vi "2_InsertQueue.vi"(6 "插入方向":enum16{"Behind", "Before"}(ring), 8 "error in (no error)":errorcluster caption="错误输入（无错误）", 9 "Data":cluster{"Cmd":T1, "Data":variant}, 10 "QueueName":T2, 11 "Queue In":refnum<queue>[](array[refnum])) -> (0 "error out":errorcluster caption="错误输出", 3 "QueueOut":refnum<queue>[](array[refnum]))   [LabVIEW 2017]
uses:
  Ctrls/QueueDataForm.ctl
  Ctrls/QueueName.ctl
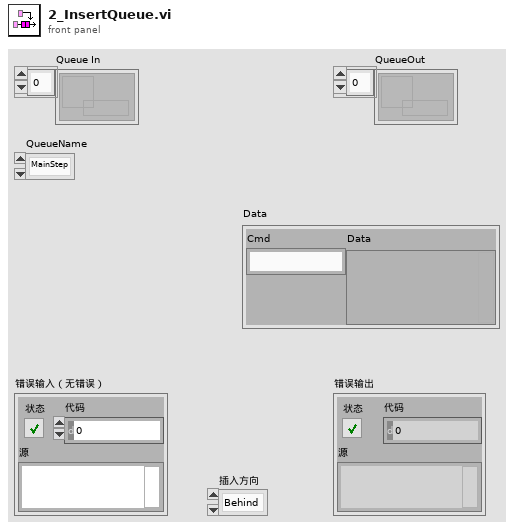
[diagram p1: front panel]
types:
  T1 = typedef "QueueDataForm.ctl" = string
  T2 = typedef "QueueName.ctl" = enum16{"MainStep", "AutoRun", "胶高"}
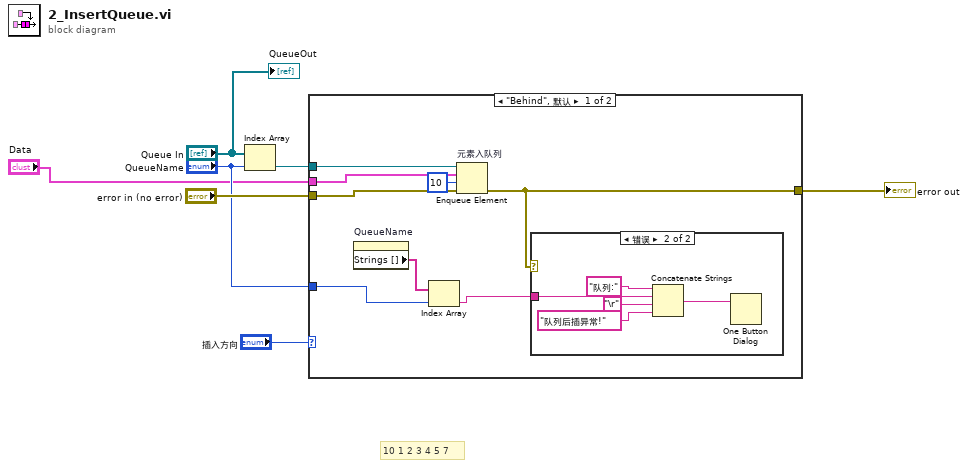
[diagram p0: block diagram]
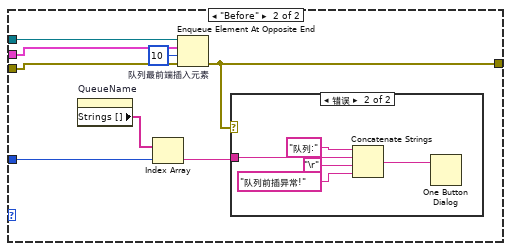
[diagram p3: hidden frame]
diagram:
  # "10 1 2 3 4 5 7"
  n1 = Index Array(array="Queue In", index="QueueName") -> (element=w6:refnum<queue>)
  n2 = case shown="\"Behind\", 默认" "插入方向" {
    tunnel: w6 -> [w15 w28]
    tunnel: "error in (no error)" -> [w14 w26]
    tunnel: "Data" -> [w13 w27]
    tunnel: [w11 w24] -> w3
    tunnel: "QueueName" -> [w9 w22]
    frame "Behind", Default {
      n3 = property on="QueueName" class="Enum (严格)"() -> ("Strings []"=w10:string[])  [unwired: 2 in, 2 out]
      n4 = Index Array(array=w10, index=w9) -> (element=w8:string)
      n5 = Enqueue Element "元素入队列"(queue=w15, element=w13, timeout in ms (-1)=10 ("超时毫秒(-1)"), error in (no error)=w14) -> (error out=w11:errorcluster)  [unwired: 2 out]
      n6 = case shown="错误" w11 {
        tunnel: w8 -> [_ w19]
        frame No Error {
        }
        frame Error {
          n7 = Concatenate Strings("队列:", w19, "\r", "队列后插异常!" ("字符串")) -> (w16:string)
          n8 = One Button Dialog(message=w16) -> ()  [unwired: 1 in, 1 out]
        }
      }
    }
    frame "Before" {
      n9 = property on="QueueName" class="Enum (严格)"() -> ("Strings []"=w23:string[])  [unwired: 2 in, 2 out]
      n10 = Index Array(array=w23, index=w22) -> (element=w21:string)
      n11 = Enqueue Element At Opposite End "队列最前端插入元素"(queue=w28, element=w27, timeout in ms (-1)=10 ("超时毫秒(-1)"), error in (no error)=w26) -> (error out=w24:errorcluster)  [unwired: 2 out]
      n12 = case shown="错误" w24 {
        tunnel: w21 -> [_ w32]
        frame No Error {
        }
        frame Error {
          n13 = Concatenate Strings("队列:", w32, "\r", "队列前插异常!" ("字符串")) -> (w29:string)
          n14 = One Button Dialog(message=w29) -> ()  [unwired: 1 in, 1 out]
        }
      }
    }
  }
  "error out" <- w3
  "QueueOut" <- "Queue In"
